vi "ActionVIOnCompile.vi"(8 "error in (no error)":errorcluster, 11 "Device Item Ref in":T1 format="%.0x") -> (0 "error out":errorcluster)   [LabVIEW 2020, in "Routing and Faulting System Explorer.lvlib"]
uses:
  Routing and Faulting System Explorer.lvlib
  <vilib>/NI VeriStand/Custom Device API/Custom Device Item Ref.ctl
  Shared/Compiled.Settings.ctl
  Shared/Communication Configuration.ctl
  Shared/Routing and Faulting Configuration.ctl
  Shared/Routing Channel Configuration.ctl
  Shared/Value-Connections Map.ctl
  Shared/Alias Mapping.ctl
  Shared/Alias Endpoint.ctl
  Shared/Compiled Connection.ctl
  Shared/FIFO Indices.ctl
  Shared/Constants.vi
  Get Channel Data in By Channel ID.vi
  <vilib>/NI VeriStand/Custom Device API/Set Item Property (Variant).vi
  <vilib>/NI VeriStand/Custom Device API/Custom Device API.lvlib
  Shared/Routing and Faulting Shared.lvlib
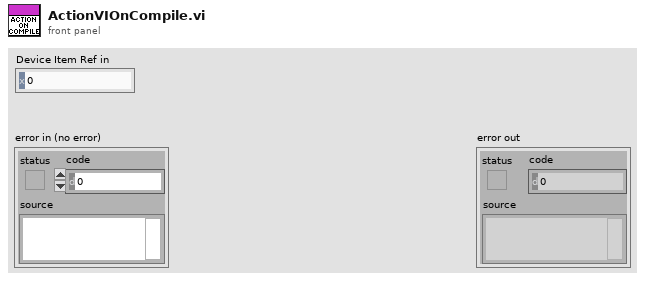
[diagram p1: front panel]
types:
  T1 = typedef "Custom Device API.lvlib/Custom Device Item Ref.ctl" = u64
  T2 = typedef "Routing and Faulting Shared.lvlib/Compiled.Settings.ctl" = cluster{"Custom Device Name":string, "Communication Configuration":T3, "Routing and Faulting Configuration":T4, "Status Channels FIFO Indices":T10}
  T3 = typedef "Routing and Faulting Shared.lvlib/Communication Configuration.ctl" = cluster{"Consumer Queue Names":string[]}
  T4 = typedef "Routing and Faulting Shared.lvlib/Routing and Faulting Configuration.ctl" = cluster{"Routing Channel Configurations":T5[], "Alias Mappings":T7[], "Compiled Connection Buffer":T9[], "Compiled Initial Connection Indices":i32[]}
  T5 = typedef "Routing and Faulting Shared.lvlib/Routing Channel Configuration.ctl" = cluster{"Channel Name":string, "Initial Value":dbl, "FIFO Index":i32, "Value-Connections Map":T6}
  T6 = typedef "Routing and Faulting Shared.lvlib/Value-Connections Map.ctl" = cluster{"State Value Array":i32[], "Connection List Array":cluster{"Compiled Connections Indices":i32[]}[]}
  T7 = typedef "Routing and Faulting Shared.lvlib/Alias Mapping.ctl" = cluster{"Alias":string, "Endpoint":T8}
  T8 = typedef "Routing and Faulting Shared.lvlib/Alias Endpoint.ctl" = cluster{"Module Path":string, "Endpoint":string}
  T9 = typedef "Routing and Faulting Shared.lvlib/Compiled Connection.ctl" = cluster{"Consumer Queue Index":i32, "Normalized Connection String":string}
  T10 = typedef "Routing and Faulting Shared.lvlib/FIFO Indices.ctl" = cluster{"Status Channel":i32, "Heartbeat Channel":i32}
  T11 = typedef "Custom Device API.lvlib/Custom Device Item Info.ctl" = cluster{"Name":string, "Is Channel":bool, "GUID":string, "Is Waveform":bool}
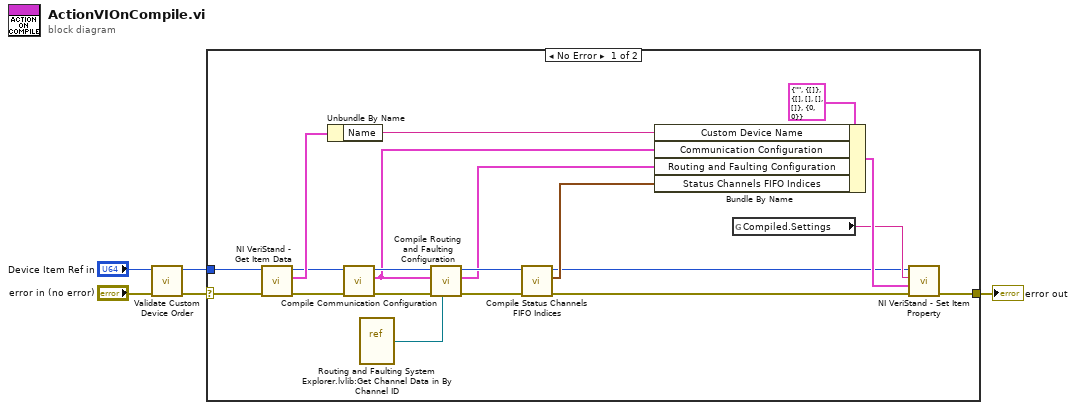
[diagram p0: block diagram]
diagram:
  n1 = call "Validate Custom Device Order.vi"("error in (no error)"="error in (no error)", "Device Item Ref in"="Device Item Ref in") -> ("error out"=w3:errorcluster, "Device Item Ref out"=w1:T1)  [unwired: 8 in]
  n2 = case shown="No Error" w3 {
    selector: w3 -> [w23 w26]
    tunnel: [w24 w26] -> w5
    tunnel: w1 -> [w22 _]
    frame No Error {
      n3 = call <vilib>:"NI VeriStand - Get Item Data.vi"("error in (no error)"=w23, "Item Ref in"=w22) -> ("error out"=w11:errorcluster, "Item Info"=w18:T11, "Item Ref out"=w12:T1)  [unwired: 6 in, 1 out]
      n4 = Unbundle By Name(w18) -> ("Name"=w19:string)
      n5 = call "Compile Communication Configuration.vi"("error in (no error)"=w11, "Device Ref in"=w12) -> ("error out"=w10:errorcluster, "Communication Configuration"=w6:T3, "Device Ref out"=w13:T1)  [unwired: 7 in]
      n6 = vi-ref "Routing and Faulting System Explorer.lvlib:Get Channel Data in By Channel ID.vi"() -> (w17:refnum<vi>)
      n7 = call "Compile Routing and Faulting Configuration.vi"("Get Channel Data Refnum"=w17, "error in (no error)"=w10, "Communication Configuration"=w6, "Device Ref in"=w13) -> ("error out"=w9:errorcluster, "RaF Configuration"=w7:T4, "Device Ref out"=w8:T1)  [unwired: 5 in]
      n8 = call "Compile Status Channels FIFO Indices.vi"("error in (no error)"=w9, "Device Ref in"=w8) -> ("error out"=w16:errorcluster, "Status Channels FIFO Indices"=w15:T10, "Device Ref out"=w14:T1)  [unwired: 7 in]
      n9 = Bundle By Name(cluster=T2 {"Custom Device Name"="", "Communication Configuration"={"Consumer Queue Names"=[]}, "Routing and Faulting Configuration"={"Routing Channel Configurations"=[], "Alias Mappings"=[], "Compiled Connection Buffer"=[], "Compiled Initial Connection Indices"=[]}, "Status Channels FIFO Indices"={"Status Channel"=0, "Heartbeat Channel"=0}} ("Compiled.Settings.ctl"), "Custom Device Name"=w19, "Communication Configuration"=w6, "Routing and Faulting Configuration"=w7, "Status Channels FIFO Indices"=w15) -> (w25:T2)
      n10 = global read "Constants.vi" "Compiled.Settings"() -> (w20:string)
      n11 = call-poly <vilib>:"NI VeriStand - Set Item Property.vi"("error in (no error)"=w16, "Value"=w25, "Property Name"=w20, "Item Ref in"=w14) -> ("error out"=w24:errorcluster)  [unwired: 5 in, 2 out]
    }
    frame Error {
    }
  }
  "error out" <- w5
